vi "Remove Dead Short.vi"() -> ()   [LabVIEW 2015]
panel:
  out "error out":errorcluster
  in  "error in":errorcluster
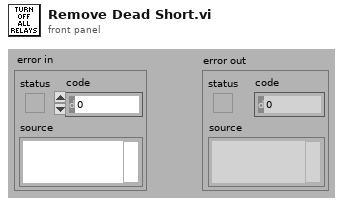
[diagram p1: front panel]
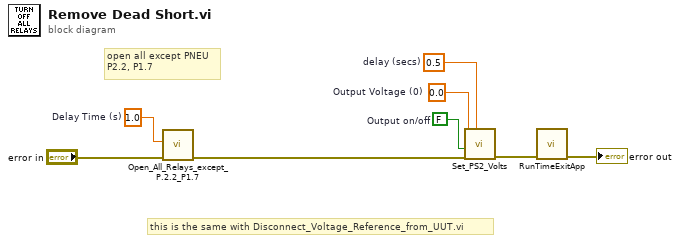
[diagram p0: block diagram]
diagram:
  w1 = 1.0  # Delay Time (s)
  w2 = FALSE  # Output on/off
  w5 = 0.5  # delay (secs)
  w6 = 0.0  # Output Voltage (0)
  # "this is the same with Disconnect_Voltage_Reference_from_UUT.vi"
  # "open all except PNEU\nP2.2, P1.7"
  n1 = call "Open_All_Relays_except_P.2.2_P1.7.vi"("Delay Time (s)"=w1, "error in"="error in") -> ("error out"=w3:errorcluster)  [unwired: 7 in]
  n2 = call "Set_PS2_Volts.vi"("delay (secs)"=w5, "error in"=w3, "Output on/off"=w2, "Output Voltage"=w6) -> ("error out"=w7:errorcluster)  [unwired: 5 in, 2 out]
  n3 = call "RunTimeExitApp.vi"("error in (no error)"=w7) -> ("error out"=→"error out":errorcluster)  [unwired: 10 in]
